vi "BoxPreRev.vi"(0 "error in":errorcluster, 11 "Boolean":bool) -> (8 "error out":errorcluster)   [LabVIEW 2023]
uses:
  <vilib>/Rock Robotics/WPI/ThirdParty/JAS_Junk/TrajLib/Trajectory_Library.lvlib
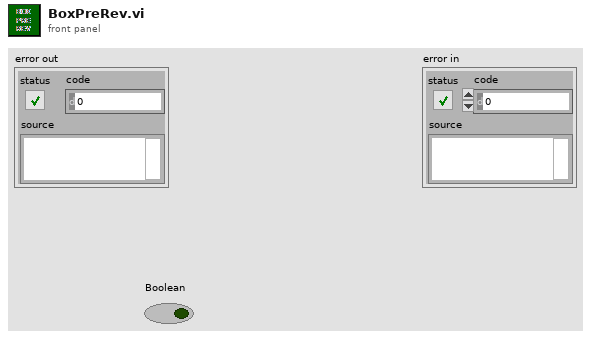
[diagram p1: front panel]
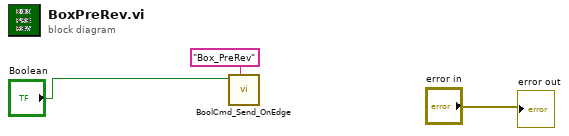
[diagram p0: block diagram]
diagram:
  n1 = call <vilib>:"BoolCmd_Send_OnEdge.vi"("Command Name"="Box_PreRev", "Value"="Boolean") -> ()  [unwired: 9 in, 1 out]
  "error out" <- "error in"
